vi "PH_AxisGUI_BaseClass.contents.vi"   [LabVIEW 2014, in "PH_AxisGUI_BaseClass.lvlib"]
doc: "This class is forseen to control motion Axes.\n\nThis class is part of the PHELIX device layer."
uses:
  PH_AxisGUI_BaseClass.lvlib
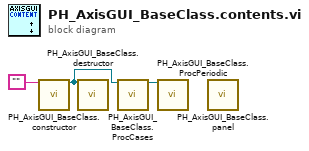
[diagram p0: block diagram]
diagram:
  n1 = call "PH_AxisGUI_BaseClass.constructor.vi"("name"="") -> ("i ref out"=w1:refnum<vi>)  [unwired: 16 in, 2 out]
  n2 = call "PH_AxisGUI_BaseClass.destructor.vi"("i ref in"=w1) -> ()  [unwired: 18 in, 1 out]
  n3 = call "PH_AxisGUI_BaseClass.ProcCases.vi"("i ref in"=w1) -> ("i ref out"=w3:refnum<vi>)  [unwired: 16 in, 2 out]
  n4 = call "PH_AxisGUI_BaseClass.ProcPeriodic.vi"("i ref in"=w3) -> ()  [unwired: 16 in, 3 out]
  n5 = call "PH_AxisGUI_BaseClass.panel.vi"() -> ()  [unwired: 19 in, 1 out]
